vi "G#Debugger_AttributeContainer.vi"(0 "MainSubPanel":refnum<vi>, 1 "VI Ref":refnum<vi>, 2 "VI Ref 2":refnum<vi>, 5 "error in (no error)":errorcluster) -> (19 "error out":errorcluster)   [LabVIEW 2017, in "G#Debugger.lvlib"]
uses:
  <vilib>/addons/_AddQ/G#Debugger/G#Debugger.lvlib
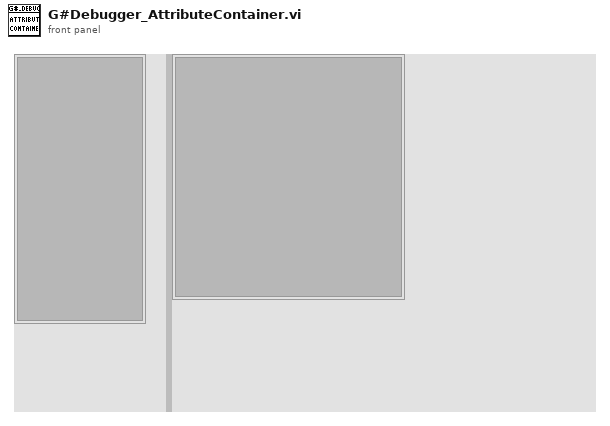
[diagram p1: front panel]
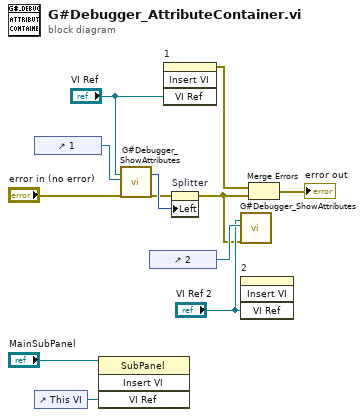
[diagram p0: block diagram]
diagram:
  n1 = control-ref of="1"() -> (w12:refnum<vi>)
  n2 = control-ref of="This VI"() -> (w4:refnum<vi>)
  n3 = invoke on="Invoke Node" class="SubPanel" method="Insert VI"(reference="MainSubPanel", "VI Ref"=w4) -> ()  [unwired: 2 in, 4 out]
  n4 = call <vilib>:"G#Debugger_ShowAttributes.vi"("VIRef"="VI Ref", "SubPanel"=w12, "error in (no error)"="error in (no error)") -> ("Width"=w3:i32, "error out"=w2:errorcluster)  [unwired: 15 in]
  n5 = control-ref of="2"() -> (w10:refnum<vi>)
  n6 = invoke on="1" class="SubPanel" method="Insert VI"("VI Ref"="VI Ref") -> (error out=w8:errorcluster)  [unwired: 3 in, 3 out]
  n7 = property on="Splitter" class="Splitter"(error in=w2, "Left"=w3) -> (error out=w1:errorcluster)  [unwired: 1 in, 1 out]
  n8 = call <vilib>:"G#Debugger_ShowAttributes.vi"("VIRef"="VI Ref 2", "SubPanel"=w10, "error in (no error)"=w1) -> ()  [unwired: 15 in, 2 out]
  n9 = invoke on="2" class="SubPanel" method="Insert VI"("VI Ref"="VI Ref 2") -> ()  [unwired: 3 in, 4 out]
  n10 = Merge Errors(w8, w1) -> (→"error out":errorcluster)
